vi "reshape debit.vi"(10 "Q":dbl[](array[numeric]), 11 "P":dbl[](array[numeric])) -> (3 "Array":dbl[](array[numeric]))   [LabVIEW 2014, in "PLS Logging.lvlib"]
uses:
  PLS Logging.lvlib
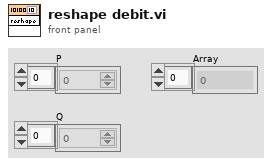
[diagram p1: front panel]
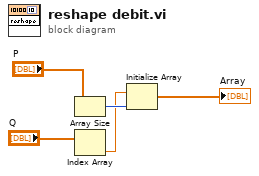
[diagram p0: block diagram]
diagram:
  n1 = Array Size(array="P") -> (size(s)=w4:i32)
  n2 = Index Array(array="Q") -> (element=w1:dbl)  [unwired: 1 in]
  n3 = Initialize Array(w1, w4) -> (→"Array":dbl[])
